vi "Param Decode KF.vi"(8 "error in (no error)":errorcluster, 10 "Array - letter":string[](array[string])) -> (0 "error out":errorcluster, 2 "Array -parameter":string[](array[string]))   [LabVIEW 2021, in "STAV lib.lvlib"]
uses:
  STAV lib.lvlib
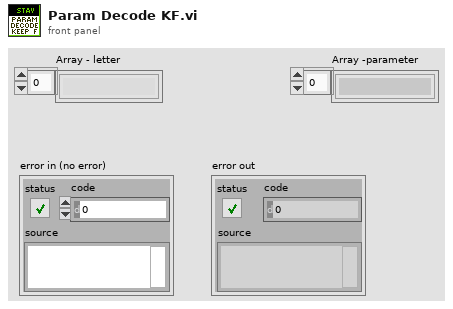
[diagram p1: front panel]
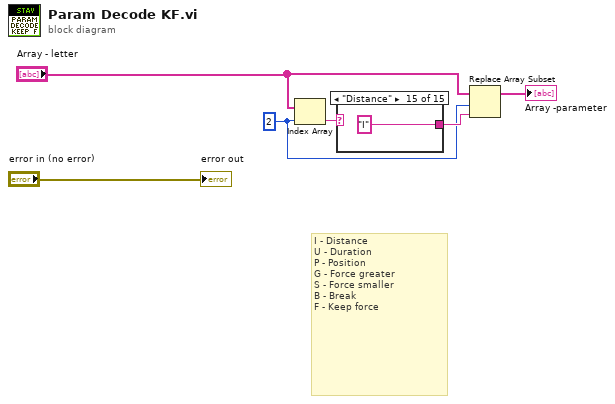
[diagram p0: block diagram]
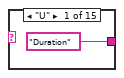
[diagram p2: hidden frame]
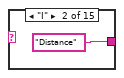
[diagram p3: hidden frame]
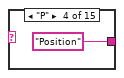
[diagram p5: hidden frame]
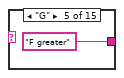
[diagram p6: hidden frame]
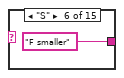
[diagram p7: hidden frame]
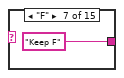
[diagram p8: hidden frame]
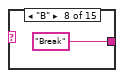
[diagram p9: hidden frame]
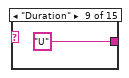
[diagram p10: hidden frame]
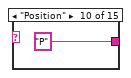
[diagram p11: hidden frame]
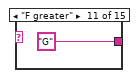
[diagram p12: hidden frame]
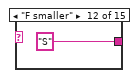
[diagram p13: hidden frame]
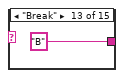
[diagram p14: hidden frame]
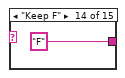
[diagram p15: hidden frame]
diagram:
  w2 = 2 ("index")
  # "I - Distance\nU - Duration\nP - Position\nG - Force greater\nS - Force smaller\nB - Break\nF - Keep force"
  n1 = Index Array(array="Array - letter", index=w2) -> (element=w1:string)
  n2 = case shown="\"Distance\"" w1 {
    selector: w1 -> [_ _ w9 _ _ _ _ _ _ _ _ _ _ _ _]
    tunnel: ["Duration" "Distance" w9 "Position" "F greater" "F smaller" "Keep F" "Break" "U" "P" "G" "S" "B" "F" "I"] -> w3
    frame "U" {
    }
    frame "I" {
    }
    frame "none", Default {
    }
    frame "P" {
    }
    frame "G" {
    }
    frame "S" {
    }
    frame "F" {
    }
    frame "B" {
    }
    frame "Duration" {
    }
    frame "Position" {
    }
    frame "F greater" {
    }
    frame "F smaller" {
    }
    frame "Break" {
    }
    frame "Keep F" {
    }
    frame "Distance" {
    }
  }
  n3 = Replace Array Subset(array="Array - letter", new element=w3, index=w2) -> (→"Array -parameter":string[])
  "error out" <- "error in (no error)"
